vi "get header items from shm clusters.vi"(7 "engine in":refnum<class "Engine Parent Editor Node.lvclass">, 8 "error in (no error)":errorcluster, 10 "shm files":T3[](array[typedef]), 11 "module editor node in":refnum<class "module editor node.lvclass">) -> (0 "error out":errorcluster, 1 "definitions":T1[](array[typedef]), 2 "structs":T2[](array[typedef]), 3 "module editor node out":refnum<class "module editor node.lvclass">, 5 "engine out":refnum<class "Engine Parent Editor Node.lvclass">)   [LabVIEW 2013, in "Shared Memory editor node.lvclass"]
uses:
  Shared Memory editor node.lvclass
  <vilib>/NI/DCAF/Tag Editor Core/Configuration Editor/Classes/Module editor node/module editor node.lvclass
  <vilib>/NI/DCAF/Tag Editor Core/Configuration Editor/Classes/Engine Parent/Engine Parent Editor Node.lvclass
  module/configuration/Memory Allocation.ctl
  module/configuration/Line.ctl
  <vilib>/NI/Tag Bus Module Framework/channel/TBM channel.lvclass
  struct params (single type).ctl
  define params.ctl
  module/configuration/Shared Memory configuration.lvclass
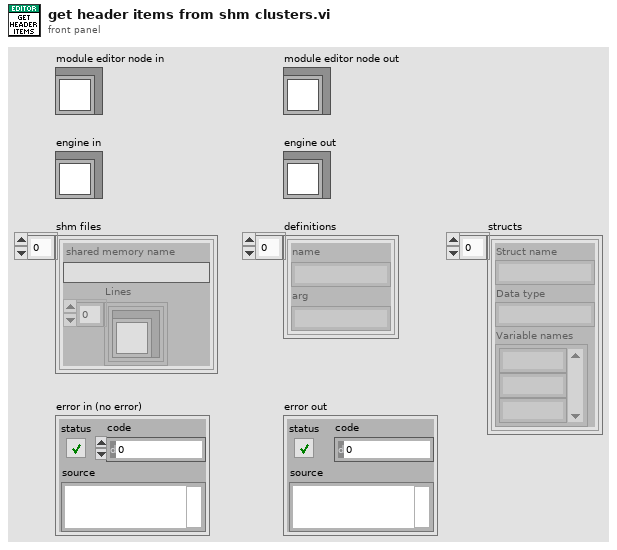
[diagram p1: front panel]
types:
  T1 = typedef "Shared Memory editor node.lvclass/define params.ctl" = cluster{"name":string, "arg":string}
  T2 = typedef "Shared Memory editor node.lvclass/struct params (single type).ctl" = cluster{"Struct name":string, "Data type":string, "Variable names":string[]}
  T3 = typedef "Shared Memory configuration.lvclass/Memory Allocation.ctl" = cluster{"shared memory name":string, "Lines":T4[]}
  T4 = typedef "Shared Memory configuration.lvclass/Line.ctl" = cluster{"channel":refnum<class "TBM channel.lvclass">}
  T5 = typedef "tag bus.lvlib/tag descriptor.lvclass/Data Type.ctl" = enum16{"Double", "Single", "I64", "I32", "I16", "I8", "U64", "U32", "U16", "U8", "Boolean", "String", "Array of Double", "Array of Single", "Array of I64", "Array of I32", "Array of I16", "Array of I8", "Array of U64", "Array of U32", "Array of U16", "Array of U8", "Array of Boolean", "Array of String"}
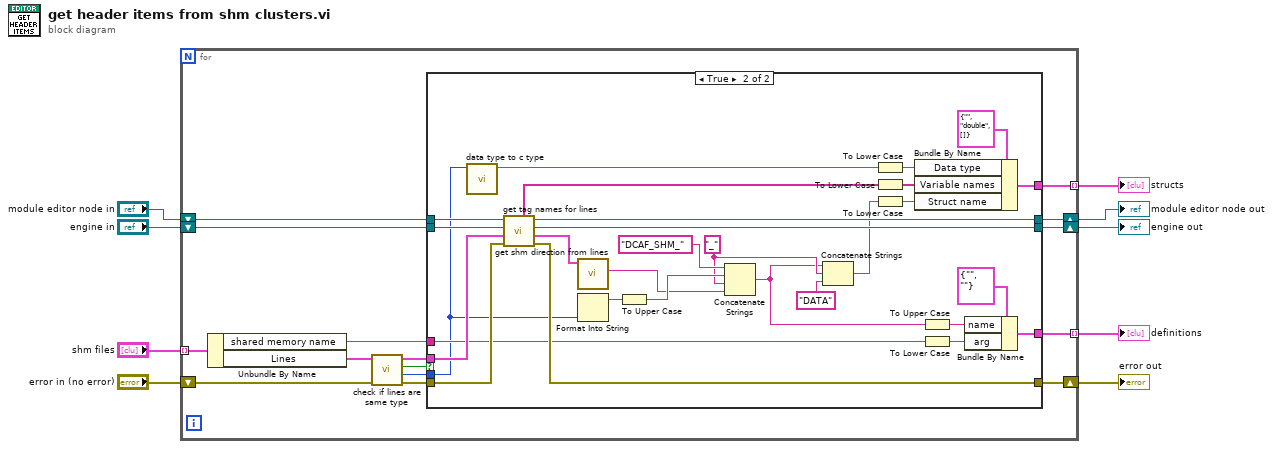
[diagram p0: block diagram]
diagram:
  n1 = for {
    tunnel: "shm files" -> [w24] mode=indexing
    shift-right: [w17] -> w8
    shift-left: "error in (no error)" -> [w18]
    shift-right: [w13] -> w7
    shift-left: "module editor node in" -> [w15]
    shift-right: [w12] -> w6
    shift-left: "engine in" -> [w14]
    tunnel: [w11] -> w2 mode=indexing
    tunnel: [w10] -> w1 mode=indexing
    n2 = Unbundle By Name(w24) -> ("shared memory name"=w16:string, "Lines"=w23:T4[])
    n3 = call "check if lines are same type.vi"("error in"=w18, "Lines in"=w23) -> ("error out"=w19:errorcluster, "type"=w20:T5, "all same type?"=w21:bool, "Lines out"=w22:T4[])  [unwired: 6 in]
    n4 = case shown="True" w21 {
      tunnel: w22 -> [_ w54]
      tunnel: w20 -> [_ w42]
      tunnel: w19 -> [w27 w48]
      tunnel: [w27 w47] -> w17
      tunnel: w16 -> [_ w46]
      tunnel: w15 -> [w25 w52]
      tunnel: w14 -> [w26 w51]
      tunnel: [w25 w50] -> w13
      tunnel: [w26 w49] -> w12
      tunnel: [_ w31] -> w11
      tunnel: [_ w30] -> w10
      frame False {
        # "Not the same type."
      }
      frame True {
        w36 = "_" ("string")
        n5 = call "data type to c type.vi"("type"=w42) -> ("c type"=w43:string)  [unwired: 10 in]
        n6 = call "get tag names for lines.vi"("error in (no error)"=w48, "Lines in"=w54, "engine in"=w51, "editor node in"=w52) -> ("error out"=w47:errorcluster, "Lines out"=w44:T4[], "engine out"=w49:refnum<class "Engine Parent Editor Node.lvclass">, "editor node out"=w50:refnum<class "module editor node.lvclass">, "tag names"=w53:string[])  [unwired: 3 in]
        n7 = call "get shm direction from lines.vi"("Lines in"=w44) -> ("direction string"=w37:string)  [unwired: 7 in, 3 out]
        n8 = Format Into String(w42) -> (resulting string=w41:string)  [unwired: 3 in, 1 out]
        n9 = To Upper Case(1:w41) -> (0:w40:string)
        n10 = Concatenate Strings("DCAF_SHM_" ("Name"), w40, w36, w37) -> (w33:string)
        n11 = Concatenate Strings(w33, w36, "DATA" ("string")) -> (w32:string)
        n12 = To Lower Case(string=w43) -> (all lower case string=w45:string)
        n13 = To Lower Case(string=w53) -> (all lower case string=w29:string[])
        n14 = To Lower Case(string=w32) -> (all lower case string=w38:string)
        n15 = Bundle By Name(cluster=T2 {"Struct name"="", "Data type"="double", "Variable names"=[]} ("struct params"), "Data type"=w45, "Variable names"=w29, "Struct name"=w38) -> (w31:T2)
        n16 = To Upper Case(1:w33) -> (0:w34:string)
        n17 = To Lower Case(string=w46) -> (all lower case string=w28:string)
        n18 = Bundle By Name(cluster=T1 {"name"="", "arg"=""} ("define params"), "name"=w34, "arg"=w28) -> (w30:T1)
      }
    }
  }
  "module editor node out" <- w7
  "engine out" <- w6
  "error out" <- w8
  "structs" <- w2
  "definitions" <- w1
